vi "Start_Stop.vi"(5 "References":T1, 6 "BD":T12 items=["Server", "Local DB"], 7 "On/Off":bool, 8 "error in":errorcluster, 9 "CtlRef":refnum<vi>, 10 "DB in":T11, 11 "PCtoMyRio in":T8={"Command"=enum."End", "Error?"=FALSE, "Stop"=FALSE, "StopPomiar"=FALSE, "Name"="", "FilesPath"=path "", "ErrorHandler"={"Threads"=enum."Acquisistion", "ClearError"=FALSE, "Error Out "={"status"=FALSE, "code"=0, "source"=""}, "Error"=FALSE}, "Fs"=0.0}) -> (0 "error out":errorcluster, 2 "DB out":T11, 3 "PCtoMyRio out":T8={"Command"=enum."End", "Error?"=FALSE, "Stop"=FALSE, "StopPomiar"=FALSE, "Name"="", "FilesPath"=path "", "ErrorHandler"={"Threads"=enum."Acquisistion", "ClearError"=FALSE, "Error Out "={"status"=FALSE, "code"=0, "source"=""}, "Error"=FALSE}, "Fs"=0.0})   [LabVIEW 2019]
uses:
  Data Saving/DataBase/TypeDef/#TypeDef_DBMode.ctl
  <vilib>/addons/database/Connection.llb/Conn ObjectReference.ctl
  Communication/TypeDef/#TypeDef_FromPCtoMR.ctl
  Communication/TypeDef/#TypeDef_Command.ctl
  Communication/TypeDef/#TypeDef_ErrorHandler_prop.ctl
  TypeDef/#TypeDef_References.ctl
  TypeDef/#TypeDef_Buttons.ctl
  TypeDef/#TypeDef_ReferencesMeassurementProp.ctl
  TypeDef/#TypeDef_ReferencesArchiveProp.ctl
  TypeDef/#TypeDef_Lists.ctl
  TypeDef/#TypeDef_MeasProp.ctl
  TypeDef/#TypeDef_OpProp.ctl
  TypeDef/#TypeDef_Enum_ModeOp.ctl
  Communication/TypeDef/#TypeDef_SetGet.ctl
  <vilib>/addons/database/NI_Database_API.lvlib
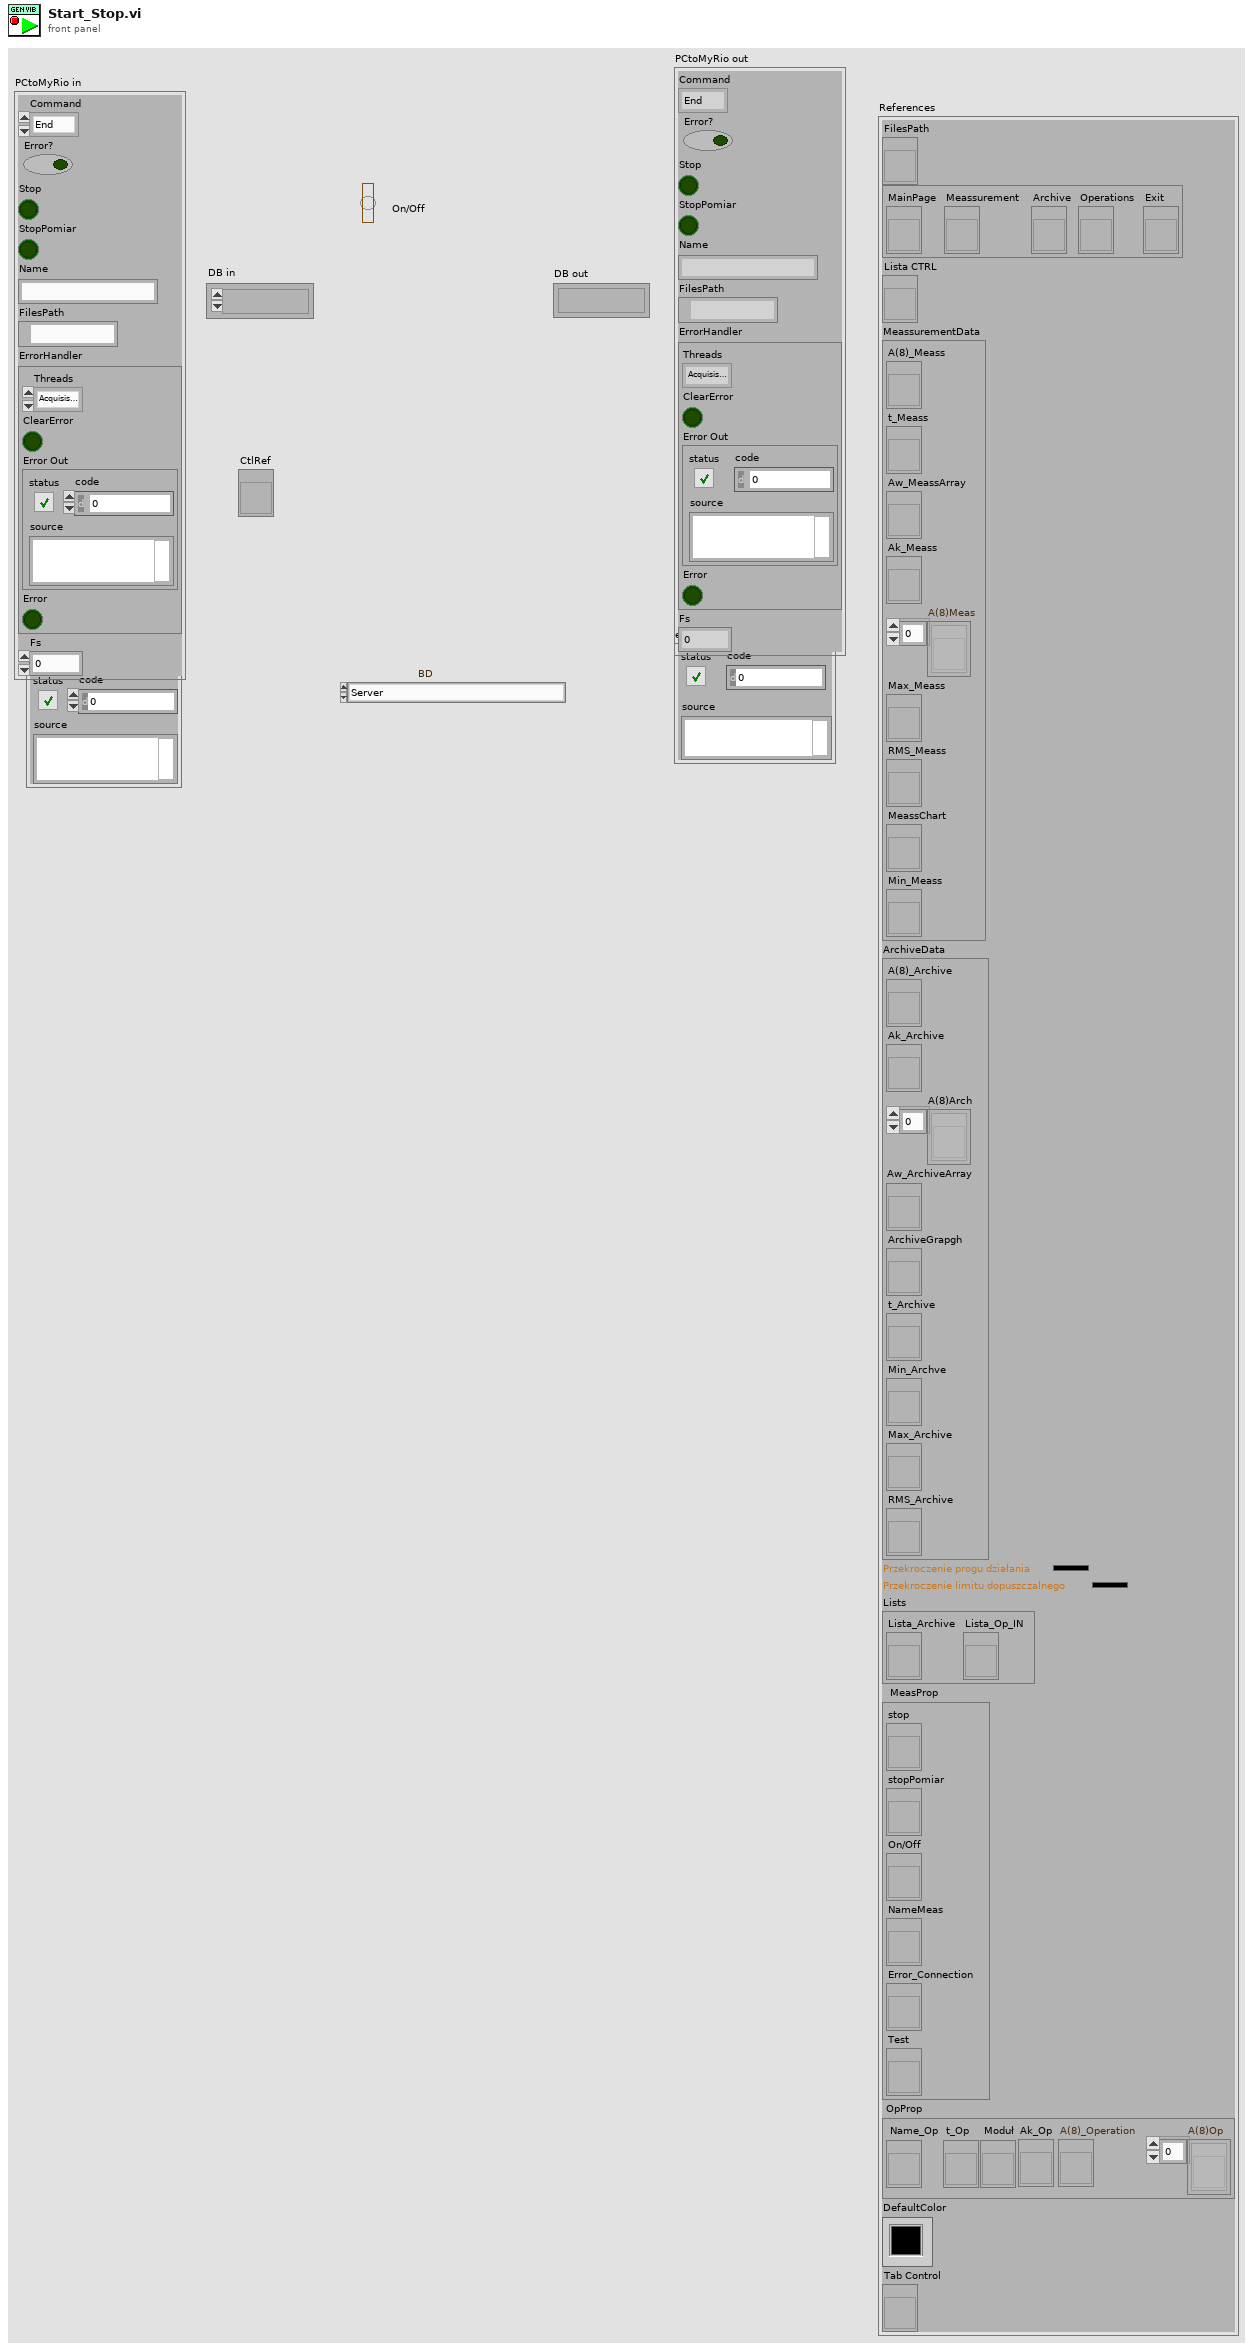
[diagram p1: front panel]
types:
  T1 = typedef "#TypeDef_References.ctl" = cluster{"FilesPath":refnum<vi>, "MainButtons":T2, "Lista CTRL":refnum<vi>, "MeassurementData":T3, "ArchiveData":T4, "PD":u32, "LD":u32, "Lists":T5, "MeasProp":T6, "OpProp":T7, "DefaultColor":u32, "Tab Control":refnum<vi>}
  T2 = typedef "#TypeDef_Buttons.ctl" = cluster{"MainPage":refnum<vi>, "Meassurement":refnum<vi>, "Archive":refnum<vi>, "Operations":refnum<vi>, "Exit":refnum<vi>}
  T3 = typedef "#TypeDef_ReferencesMeassurementProp.ctl" = cluster{"A(8)_Meass":refnum<vi>, "t_Meass":refnum<vi>, "Aw_MeassArray":refnum<vi>, "Ak_Meass":refnum<vi>, "A(8)Meas":refnum<vi>[], "Max_Meass":refnum<vi>, "RMS_Meass":refnum<vi>, "MeassChart":refnum<vi>, "Min_Meass":refnum<vi>}
  T4 = typedef "#TypeDef_ReferencesArchiveProp.ctl" = cluster{"A(8)_Archive":refnum<vi>, "Ak_Archive":refnum<vi>, "A(8)Arch":refnum<vi>[], "Aw_ArchiveArray":refnum<vi>, "ArchiveGrapgh":refnum<vi>, "t_Archive":refnum<vi>, "Min_Archve":refnum<vi>, "Max_Archive":refnum<vi>, "RMS_Archive":refnum<vi>}
  T5 = typedef "#TypeDef_Lists.ctl" = cluster{"Lista_Archive":refnum<vi>, "Lista_Op_IN":refnum<vi>}
  T6 = typedef "#TypeDef_MeasProp.ctl" = cluster{"stop":refnum<vi>, "stopPomiar":refnum<vi>, "On/Off":refnum<vi>, "NameMeas":refnum<vi>, "Error_Connection":refnum<vi>, "Test":refnum<vi>}
  T7 = typedef "#TypeDef_OpProp.ctl" = cluster{"Name_Op":refnum<vi>, "t_Op":refnum<vi>, "Modu³":refnum<vi>, "Ak_Op":refnum<vi>, "A(8)_Operation":refnum<vi>, "A(8)Op":refnum<vi>[]}
  T8 = typedef "#TypeDef_FromPCtoMR.ctl" = cluster{"Command":T9, "Error?":bool, "Stop":bool, "StopPomiar":bool, "Name":string, "FilesPath":path, "ErrorHandler":T10, "Fs":dbl}
  T9 = typedef "#TypeDef_Command.ctl" = enum16{"Start", "End"}
  T10 = typedef "#TypeDef_ErrorHandler_prop.ctl" = cluster{"Threads":enum16{"Acquisistion", "Data Operation", "Save File"}, "ClearError":bool, "Error Out ":errorcluster, "Error":bool}
  T11 = typedef "NI_Database_API.lvlib/Conn ObjectReference.ctl" = refnum<k1>
  T12 = typedef "#TypeDef_DBMode.ctl" = u16
  T13 = typedef "#TypeDef_SetGet.ctl" = enum16{"Set", "Get"}
  T14 = enum8{"Enabled", "Disabled", "Disabled and Grayed Out"}
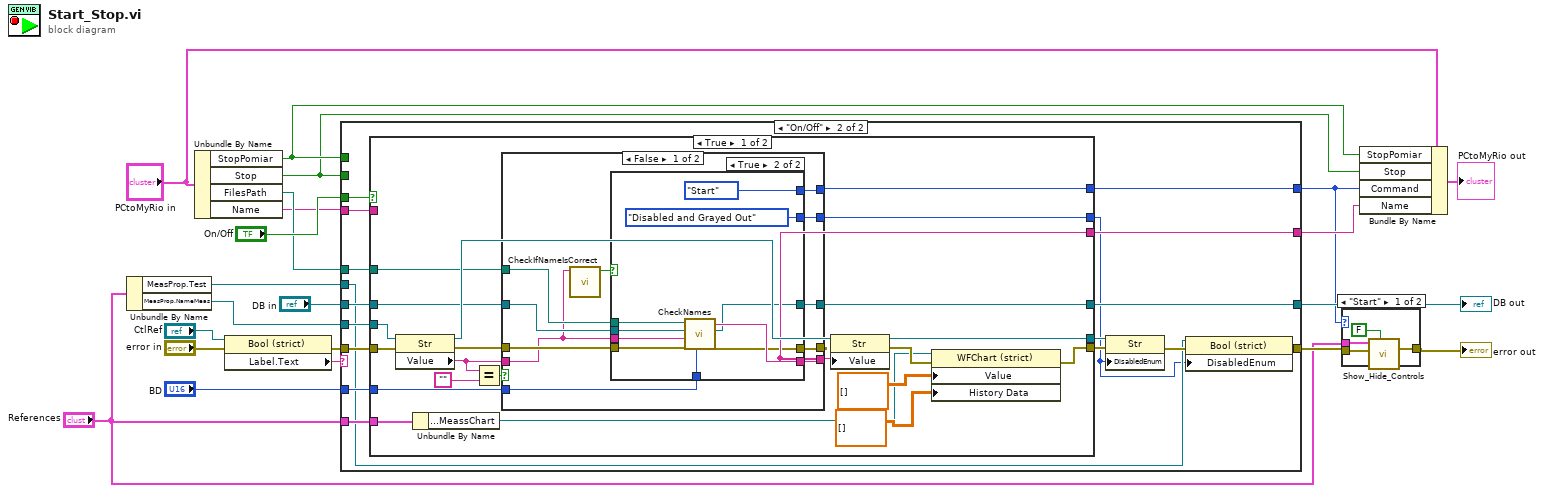
[diagram p0: block diagram]
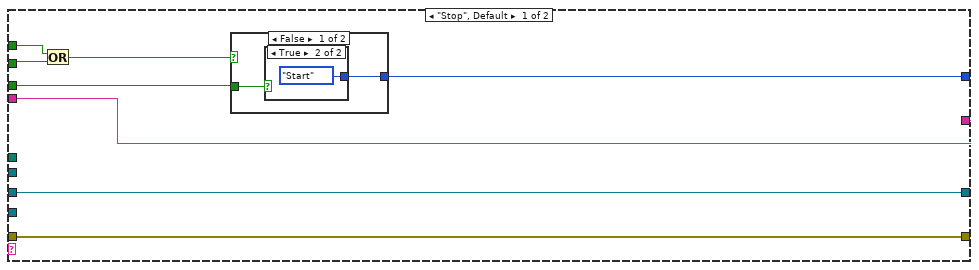
[diagram p2: hidden frame]
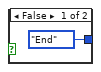
[diagram p3: hidden frame]
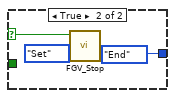
[diagram p4: hidden frame]
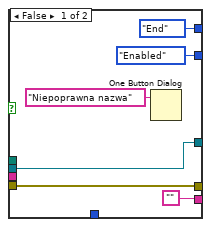
[diagram p5: hidden frame]
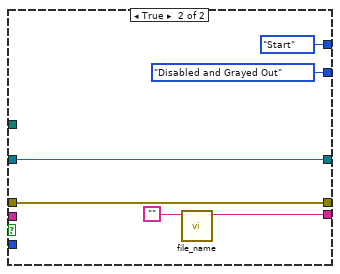
[diagram p6: hidden frame]
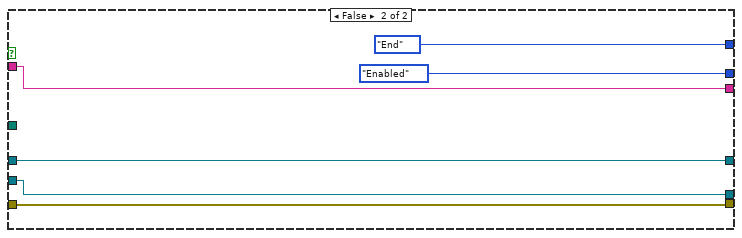
[diagram p7: hidden frame]
diagram:
  n1 = Unbundle By Name("References") -> ("MeasProp.Test"=w1:refnum<vi>, "MeasProp.NameMeas"=w4:refnum<vi>)
  n2 = Unbundle By Name("PCtoMyRio in") -> ("StopPomiar"=w13:bool, "Stop"=w11:bool, "FilesPath"=w15:path, "Name"=w7:string)
  n3 = property class="Bool (strict)"(reference="CtlRef", error in="error in") -> (error out=w18:errorcluster, "Label.Text"=w21:string)  [unwired: 1 out]
  n4 = case shown="\"On/Off\"" w21 {
    tunnel: w11 -> [w25 _]
    tunnel: "On/Off" -> [w29 w53]
    tunnel: [w28 w48] -> w5
    tunnel: w18 -> [w27 w52]
    tunnel: w4 -> [_ w49]
    tunnel: [w27 w39] -> w6
    tunnel: w15 -> [_ w51]
    tunnel: w13 -> [w26 _]
    tunnel: "BD" -> [_ w46]
    tunnel: "DB in" -> [w23 w45]
    tunnel: [w23 w44] -> w9
    tunnel: [w22 w43] -> w8
    tunnel: w7 -> [w22 w42]
    tunnel: "References" -> [_ w41]
    tunnel: w1 -> [_ w38]
    frame "Stop", Default {
      n5 = Or(x=w26, y=w25) -> (x .or. y?=w24:bool)
      n6 = case shown="False" w24 {
        selector: w24 -> [_ w35]
        tunnel: [w31 #TypeDef_Command."End" ("Command")] -> w28
        tunnel: w29 -> [w30 _]
        frame False {
          n7 = case shown="True" w30 {
            tunnel: [#TypeDef_Command."End" ("Command") #TypeDef_Command."Start" ("Command")] -> w31
            frame False {
            }
            frame True {
            }
          }
        }
        frame True {
          n8 = call "FGV_Stop.vi"("Get/Set"=#TypeDef_SetGet."Set", "STOP in"=w35) -> ()  [unwired: 9 in, 1 out]
        }
      }
    }
    frame "On/Off" {
      n9 = case shown="True" w53 {
        tunnel: [w61 T14."Enabled" ("f")] -> w37
        tunnel: [w60 #TypeDef_Command."End" ("Command")] -> w48
        tunnel: w52 -> [w71 w110]
        tunnel: w51 -> [w66 _]
        tunnel: [w67 w111] -> w50
        tunnel: w49 -> [w74 w111]
        tunnel: [w56 w110] -> w47
        tunnel: w46 -> [w65 _]
        tunnel: w45 -> [w64 w109]
        tunnel: [w63 w109] -> w44
        tunnel: [w62 w108] -> w43
        tunnel: w42 -> [_ w108]
        tunnel: w41 -> [w55 _]
        frame True {
          n10 = property class="Str"(reference=w74, error in=w71) -> (reference out=w68:refnum<vi>, error out=w73:errorcluster, "Value"=w72:string)
          n11 = Unbundle By Name(w55) -> ("MeassurementData.MeassChart"=w54:refnum<vi>)
          n12 = Equal?(x=w72, y="") -> (x = y?=w69:bool)
          n13 = case shown="False" w69 {
            tunnel: w73 -> [w84 w107]
            tunnel: [w83 w107] -> _
            tunnel: w72 -> [w76 _]
            tunnel: [w85 w105] -> w62
            tunnel: w66 -> [w82 _]
            tunnel: w65 -> [w79 _]
            tunnel: w64 -> [w81 w106]
            tunnel: [w80 w106] -> w63
            tunnel: [w78 T14."Disabled and Grayed Out" ("Disabled")] -> w61
            tunnel: [w77 #TypeDef_Command."Start" ("Command")] -> w60
            frame False {
              n14 = call "CheckIfNameIsCorrect.vi"("Name"=w76) -> ("Correct?"=w75:bool)  [unwired: 10 in]
              n15 = case shown="True" w75 {
                tunnel: w76 -> [_ w101]
                tunnel: ["" w100] -> w85
                tunnel: w84 -> [w90 w99]
                tunnel: [w90 w98] -> w83
                tunnel: w82 -> [_ w97]
                tunnel: w81 -> [w91 w96]
                tunnel: [w91 w95] -> w80
                tunnel: w79 -> [_ w94]
                tunnel: [T14."Enabled" ("Disabled") T14."Disabled and Grayed Out" ("Disabled")] -> w78
                tunnel: [#TypeDef_Command."End" ("Command") #TypeDef_Command."Start" ("Command")] -> w77
                frame False {
                  n16 = One Button Dialog(message="Niepoprawna nazwa") -> ()  [unwired: 1 in, 1 out]
                }
                frame True {
                  n17 = call "CheckNames.vi"("BD"=w94, "error in"=w99, "Value in"=w101, "DB in"=w96, "Path"=w97) -> ("error out"=w98:errorcluster, "DB out"=w95:T11, "Value out"=w100:string)  [unwired: 4 in]
                }
              }
            }
            frame True {
              n18 = call "file_name.vi"("String in"="") -> ("String out"=w105:string)  [unwired: 8 in]
            }
          }
          n19 = property class="Str"(reference=w68, "Value"=w62) -> (reference out=w67:refnum<vi>, error out=w57:errorcluster)  [unwired: 1 in]
          n20 = property class="WFChart (strict)"(reference=w54, error in=w57, "Value"=dbl[][] [], "History Data"=dbl[][] []) -> (error out=w56:errorcluster)  [unwired: 1 out]
        }
        frame False {
        }
      }
      n21 = property class="Str"(reference=w50, error in=w47, "DisabledEnum"=w37) -> (error out=w40:errorcluster)  [unwired: 1 out]
      n22 = property class="Bool (strict)"(reference=w38, error in=w40, "DisabledEnum"=w37) -> (error out=w39:errorcluster)  [unwired: 1 out]
    }
  }
  "DB out" <- w9
  n23 = case shown="\"Start\"" w5 {
    tunnel: "References" -> [w116 _]
    tunnel: w6 -> [w115 w118]
    tunnel: [w114 w118] -> w2
    frame "Start" {
      n24 = call "Show_Hide_Controls.vi"("Visible"=FALSE, "error in"=w115, "References"=w116) -> ("error out"=w114:errorcluster)  [unwired: 8 in]
    }
    frame "End", Default {
    }
  }
  "error out" <- w2
  n25 = Bundle By Name(cluster="PCtoMyRio in", "StopPomiar"=w13, "Stop"=w11, "Command"=w5, "Name"=w8) -> (→"PCtoMyRio out":T8)
